vi "add_line_enface_IMAQ.vi"(6 "Output Line":i32, 8 "error in (no error)":errorcluster, 9 "Input Line":dbl=74.0, 10 "Raw Image":T1, 11 "En Face Image":T1) -> (0 "error out":errorcluster, 3 "En Face Image Out":T1)   [LabVIEW 2016]
uses:
  <vilib>/vision/Image Controls.llb/IMAQ Image.ctl
  <vilib>/vision/NI_Vision_Development_Module.lvlib
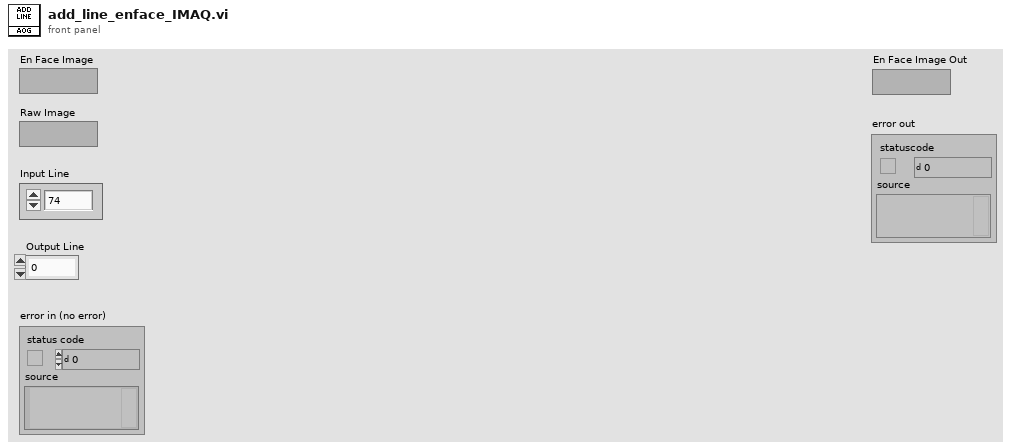
[diagram p1: front panel]
types:
  T1 = typedef "IMAQ Image.ctl" = refnum<image>
  T2 = typedef "Image Type" = u32
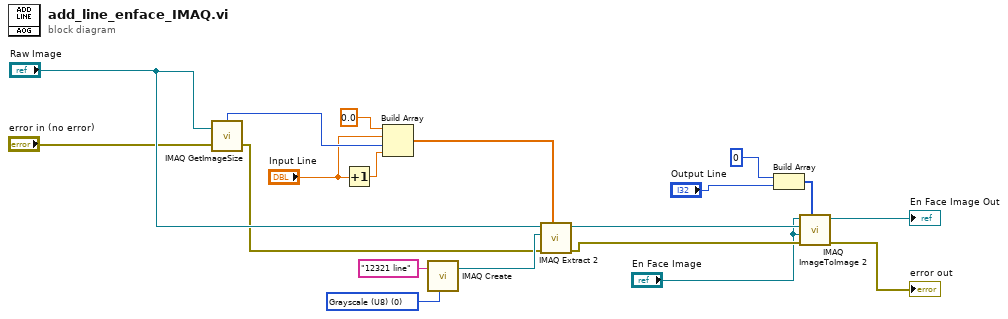
[diagram p0: block diagram]
diagram:
  w17 = T2 0 items=["Grayscale (U8)", "Grayscale (I16)", "Grayscale (SGL)", "Complex (CSG)", "RGB (U32)", "HSL (U32)", "RGB (U64)", "Grayscale (U16)"] ("Image Type")
  n1 = call "IMAQ GetImageSize"("Image"="Raw Image", "error in (no error)"="error in (no error)") -> ("X Resolution"=w4:i32, "error out"=w5:errorcluster)  [unwired: 2 in, 1 out]
  n2 = Increment(x="Input Line") -> (x+1=w2:dbl)
  n3 = Build Array(0.0 ("element"), "Input Line", w4, w2) -> (w15:dbl[])
  n4 = call "IMAQ Create"("Image Name"="12321 line", "Image Type"=w17) -> ("New Image"=w16:T1)  [unwired: 3 in, 1 out]
  n5 = call "IMAQ Extract 2"("Optional Rectangle"=w15, "error in (no error)"=w5, "Image Dst"=w16, "Image Src"="Raw Image") -> ("error out"=w6:errorcluster, "Image Dst Out"=w14:T1)  [unwired: 6 in]
  n6 = Build Array(0 ("element"), "Output Line") -> (w10:i32[])
  n7 = call "IMAQ ImageToImage 2"("Offset Left/Top"=w10, "error in (no error)"=w6, "Image Dst"="En Face Image", "Image Src (Small)"=w14, "Image Src (Large)"="En Face Image") -> ("error out"=→"error out":errorcluster, "Image Dst Out"=→"En Face Image Out":T1)  [unwired: 5 in]
